vi "LoopSpeedTester.vi"() -> ()   [LabVIEW 2023]
panel:
  out "LabJack Error":errorcluster
  out "UD Backlog [%]":dbl format="%.2f"
  out "Comm Backlog [%]":dbl format="%.2f"
  out "# Scans Read":i32
  in  "Res Index":dbl
  in  "# Channels":i32=4
  in  "Scans To Read Per Iteration":dbl=1.0 format="%.3f"
  out "Actual Scan Rate (Hz)":dbl format="%.3f"
  in  "Scan Rate (Hz)":dbl=10.0 format="%.3f"
  out "?":bool
  in  "?":bool
  out "Delimited Spreadsheet Error":errorcluster
  out "File Error":errorcluster
  in  "Path":path
  out "Full filepath":string
  in  "File extension":string
  in  "Filename":string
  out "Time Stamp":timestamp
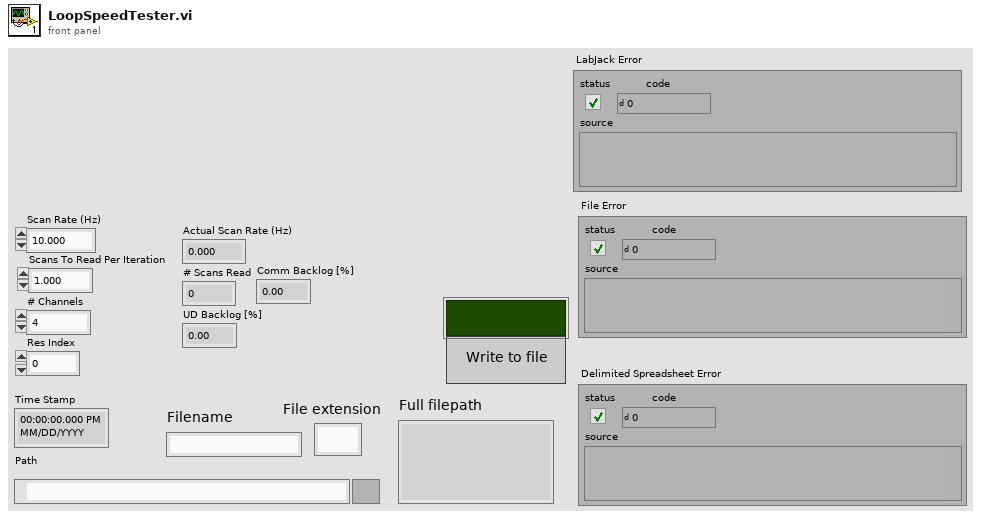
[diagram p1: front panel]
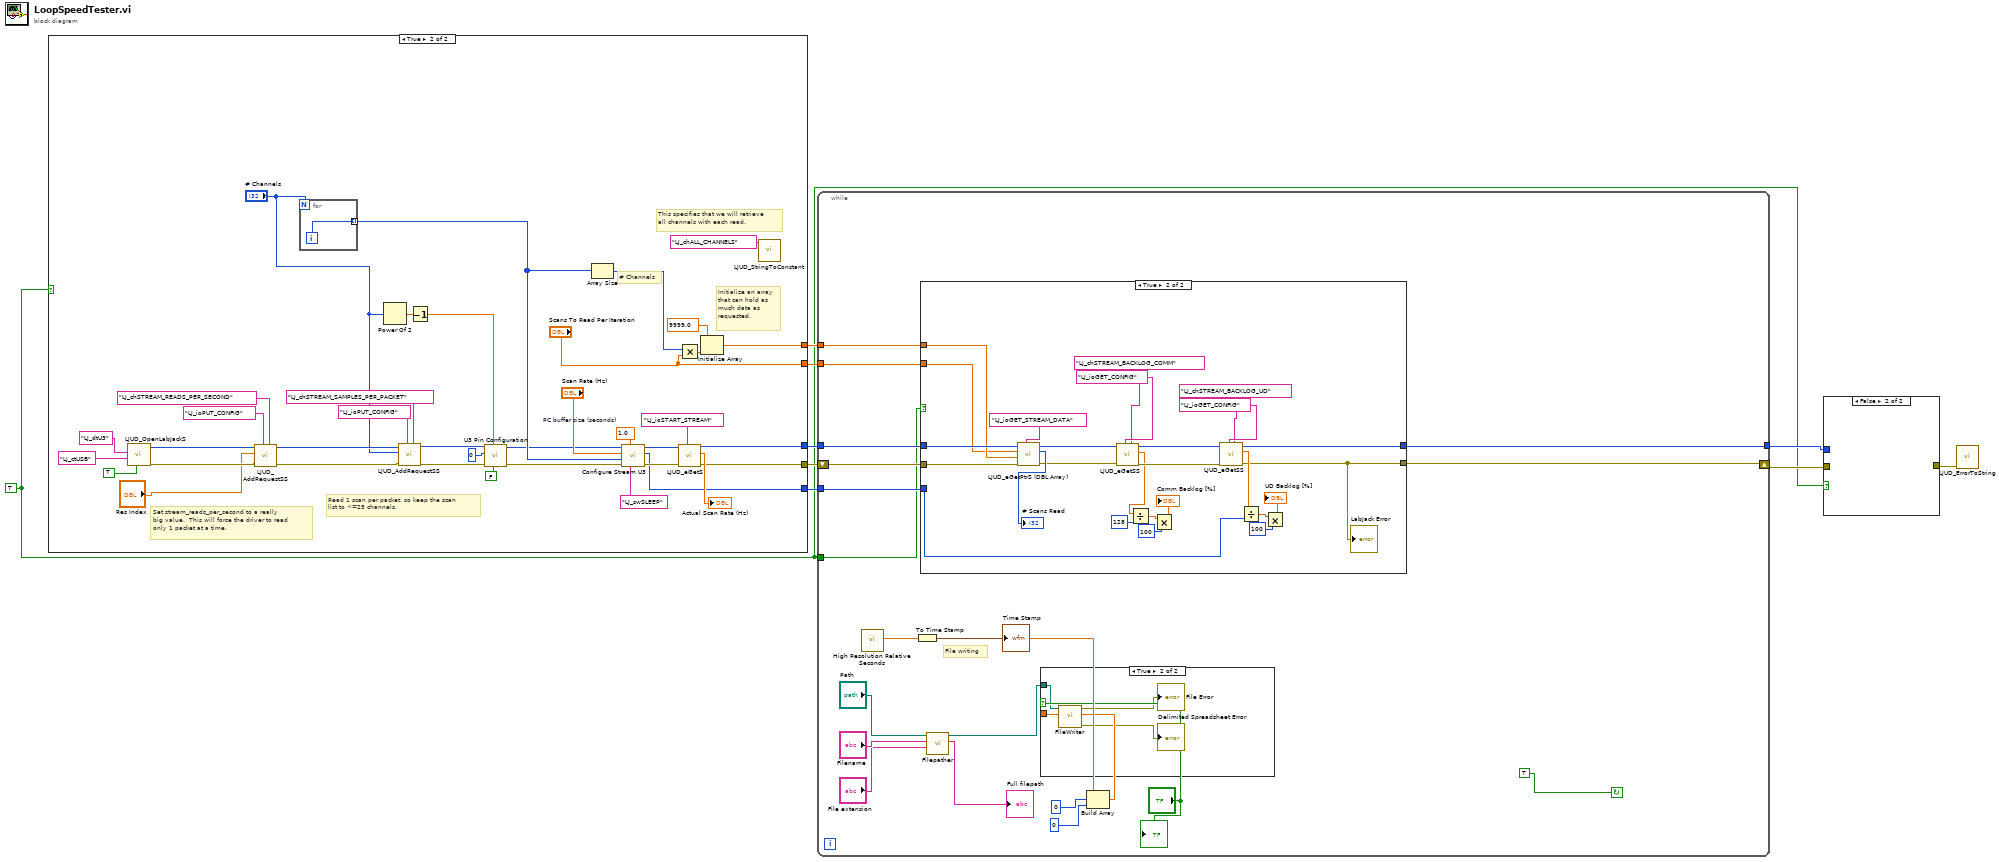
[diagram p0: block diagram]
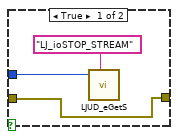
[diagram p2: hidden frame]
diagram:
  w1 = TRUE
  n1 = case shown="True" w1 {
    tunnel: [_ w14] -> w9
    tunnel: [_ w13] -> w8
    tunnel: [_ w12] -> w4
    tunnel: [_ w11] -> w3
    tunnel: [_ "Scans To Read Per Iteration"] -> w2
    frame False {
    }
    frame True {
      w26 = 1.0  # PC buffer size (seconds)
      # "Set stream_reads_per_second to a really\nbig value.  This will force the driver to read\nonly 1 packet at a time."
      # "Read 1 scan per packet, so keep the scan\nlist to <=25 channels."
      # "Initialize an array\nthat can hold as\nmuch data as\nrequested."
      # "# Channels"
      # "This specifies that we will retrieve\nall channels with each read."
      n2 = call <vilib>:"LJUD_OpenLabJackS.vi"("FirstFound"=TRUE, "ConnectionType"="LJ_ctUSB", "DeviceType"="LJ_dtU3") -> ("error out"=w28:errorcluster, "Handle"=w30:i32)  [unwired: 6 in, 1 out]
      n3 = call <vilib>:"LJUD_AddRequestSS.vi"("Channel"="LJ_chSTREAM_READS_PER_SECOND" ("IOType"), "IOType"="LJ_ioPUT_CONFIG", "error in"=w28, "Value"="Res Index", "Handle In"=w30) -> ("error out"=w27:errorcluster, "Handle Out"=w29:i32)  [unwired: 5 in]
      n4 = for {
        N: "# Channels" -> [_]
        tunnel: [w48] -> w25 mode=indexing
        i -> [w48]
      }
      n5 = Power Of 2(x="# Channels") -> (2^x=w17:dbl)
      n6 = call <vilib>:"LJUD_AddRequestSS.vi"("Channel"="LJ_chSTREAM_SAMPLES_PER_PACKET" ("IOType"), "IOType"="LJ_ioPUT_CONFIG", "error in"=w27, "Value"="# Channels", "Handle In"=w29) -> ("error out"=w24:errorcluster, "Handle Out"=w22:i32)  [unwired: 5 in]
      n7 = Decrement(x=w17) -> (x-1=w16:dbl)
      n8 = call <vilib>:"U3 Pin Configuration.vi"("Enable Counter0"=FALSE, "FIO/EIO Analog Enable"=w16, "error in"=w24, "Number of Timers Enabled"=u8 0, "Handle In"=w22) -> ("error out"=w23:errorcluster, "Handle Out"=w21:i32)  [unwired: 5 in]
      n9 = Array Size(array=w25) -> (size(s)=w42:i32)
      n10 = call <vilib>:"Configure Stream U3.vi"("Wait Mode"="LJ_swSLEEP" ("Wait Mode (2)"), "PC buffer size (seconds)"=w26, "error in"=w23, "Scan List (+)"=w25, "Scan Rate (Hz)"="Scan Rate (Hz)", "Handle In"=w21) -> ("error out"=w45:errorcluster, "PC buffer size (samples)"=w12:i32, "Handle Out"=w46:i32)  [unwired: 3 in]
      n11 = Multiply(x=w42, y="Scans To Read Per Iteration") -> (x*y=w44:dbl)
      n12 = call <vilib>:"LJUD_eGetS.vi"("IOType"="LJ_ioSTART_STREAM", "error in"=w45, "Handle In"=w46) -> ("error out"=w14:errorcluster, "Value Read"=→"Actual Scan Rate (Hz)":dbl, "Handle Out"=w13:i32)  [unwired: 6 in]
      n13 = Initialize Array(9999.0, w44) -> (w11:dbl[])
      n14 = call <vilib>:"LJUD_StringToConstant.vi"("String"="LJ_chALL_CHANNELS") -> ()  [unwired: 9 in, 2 out]
    }
  }
  n15 = while {
    shift-right: [w55] -> w6
    shift-left: w9 -> [w56]
    tunnel: w8 -> [w54]
    tunnel: [w53] -> w5
    tunnel: w4 -> [w52]
    tunnel: w3 -> [w51]
    tunnel: w2 -> [w50]
    tunnel: w1 -> [w49]
    stop <- TRUE continue-if-true
    # "File writing"
    n16 = call <vilib>:"High Resolution Relative Seconds.vi"() -> ("relative seconds"=w64:dbl)
    n17 = To Time Stamp(1:w64) -> (0:→"Time Stamp":timestamp)
    n18 = case shown="True" w49 {
      tunnel: w56 -> [_ w81]
      tunnel: [_ w69] -> w55
      tunnel: w54 -> [_ w77]
      tunnel: [_ w74] -> w53
      tunnel: w52 -> [_ w72]
      tunnel: w51 -> [_ w71]
      tunnel: w50 -> [_ w70]
      frame False {
      }
      frame True {
        n19 = call <vilib>:"LJUD_eGetPtrS (DBL Array).vi"("IOType"="LJ_ioGET_STREAM_DATA", "error in"=w81, "DBL Array Write"=w71, "Value"=w70, "Handle In"=w77) -> ("error out"=w80:errorcluster, "Value"=→"# Scans Read":i32, "Handle Out"=w76:i32)  [unwired: 3 in, 1 out]
        n20 = call <vilib>:"LJUD_eGetSS.vi"("Channel"="LJ_chSTREAM_BACKLOG_COMM", "IOType"="LJ_ioGET_CONFIG", "error in"=w80, "Handle In"=w76) -> ("error out"=w79:errorcluster, "Value Read"=w78:dbl, "Handle Out"=w75:i32)  [unwired: 5 in]
        n21 = Divide(x=w78, y=128) -> (x/y=w90:dbl)
        n22 = Multiply(x=w90, y=100) -> (x*y=→"Comm Backlog [%]":dbl)
        n23 = call <vilib>:"LJUD_eGetSS.vi"("Channel"="LJ_chSTREAM_BACKLOG_UD", "IOType"="LJ_ioGET_CONFIG", "error in"=w79, "Handle In"=w75) -> ("error out"=w69:errorcluster, "Value Read"=w73:dbl, "Handle Out"=w74:i32)  [unwired: 5 in]
        "LabJack Error" <- w69
        n24 = Divide(x=w73, y=w72) -> (x/y=w93:dbl)
        n25 = Multiply(x=w93, y=100) -> (x*y=→"UD Backlog [%]":dbl)
      }
    }
    n26 = call "Filepather.vi"("File extension"="File extension", "Filename"="Filename", "Path in"="Path") -> ("Full filepath"=→"Full filepath":string, "Path out"=w57:path)  [unwired: 7 in]
    n27 = Build Array(w64, 0, 0) -> (w63:dbl[])
    n28 = case shown="True" "?" {
      tunnel: w63 -> [_ w96]
      tunnel: w57 -> [_ w95]
      frame False {
      }
      frame True {
        n29 = call "FileWriter.vi"("Array"=w96, "Path in"=w95) -> ("Delimited Conversion Error"=→"Delimited Spreadsheet Error":errorcluster, "File Error"=→"File Error":errorcluster)  [unwired: 8 in]
      }
    }
    "?" <- "?"
  }
  n30 = case shown="False" w1 {
    tunnel: w5 -> [w100 _]
    tunnel: [w99 _] -> w7
    tunnel: w6 -> [w99 _]
    frame True {
      n31 = call <vilib>:"LJUD_eGetS.vi"("IOType"="LJ_ioSTOP_STREAM", "Handle In"=w100) -> ()  [unwired: 7 in, 3 out]
    }
    frame False {
    }
  }
  n32 = call <vilib>:"LJUD_ErrorToString.vi"("error in"=w7) -> ()  [unwired: 10 in, 1 out]
